vi "LoadControlPanel.vi"(8 "error in (no error)":errorcluster, 10 "Actor In":refnum<class "Actor.lvclass">, 11 "Microscope in":refnum<class "Microscope.lvclass">) -> (0 "error out":errorcluster, 3 "Microscope out":refnum<class "Microscope.lvclass">)   [LabVIEW 2020, in "Microscope.lvlib" / "Microscope.lvclass"]
uses:
  Microscope.lvclass
  <vilib>/ActorFramework/Actor/Actor.lvclass
  Component/Device/Device/DataExchange.ctl
  ViewController/Microscope Controller/MicroscopeController.lvclass
  C:/Program Files/National Instruments/LabVIEW 2020/vi.lib/ActorFramework/Actor/Actor.lvclass
  Microscope.lvclass/Microscope.ctl
  Interface/DataListener Messages/OnDataChange Msg/OnDataChange Msg.lvclass/OnDataChange Msg.ctl
  <vilib>/ActorFramework/Message Enqueuer/Message Enqueuer.lvclass/Message Enqueuer.ctl
  <vilib>/ActorFramework/Message Enqueuer/Enqueue.vi
  Interface/DataListener Messages/OnDataChange Msg/OnDataChange Msg.lvclass
  C:/Program Files/National Instruments/LabVIEW 2020/vi.lib/ActorFramework/Message/Message.lvclass
  <vilib>/ActorFramework/Message Priority Queue/Priority Enqueue.vi
  Component/Device/Device/Device.lvclass
  Interface/DataListener/DataListener.lvclass
panel:
  in  "cluster":T1
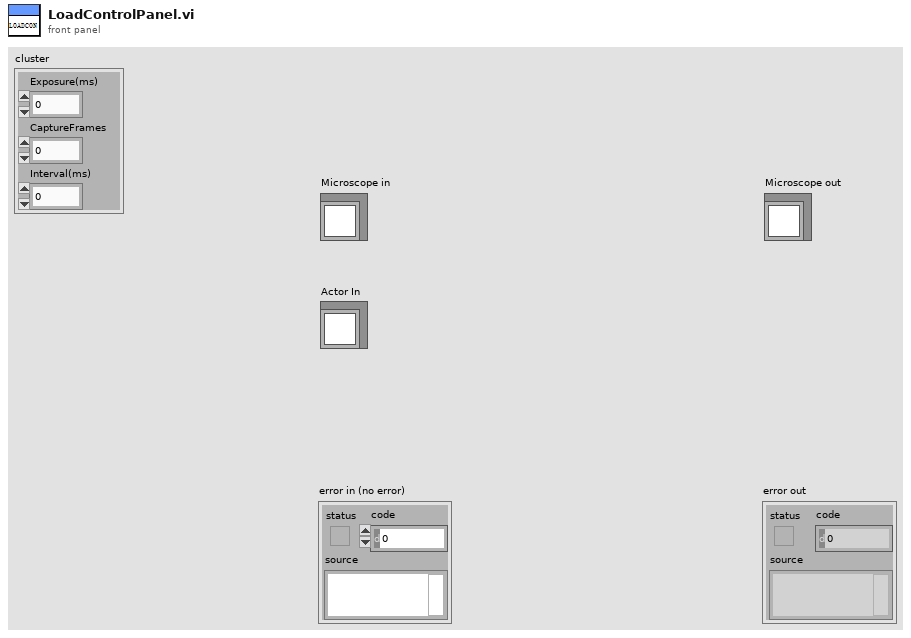
[diagram p1: front panel]
types:
  T1 = cluster{"Exposure(ms)":dbl, "CaptureFrames":dbl, "Interval(ms)":dbl}
  T2 = typedef "DataListener.lvclass/DataExchange.ctl" = cluster{"Source":string, "Destination":string, "Description":string, "value":variant}
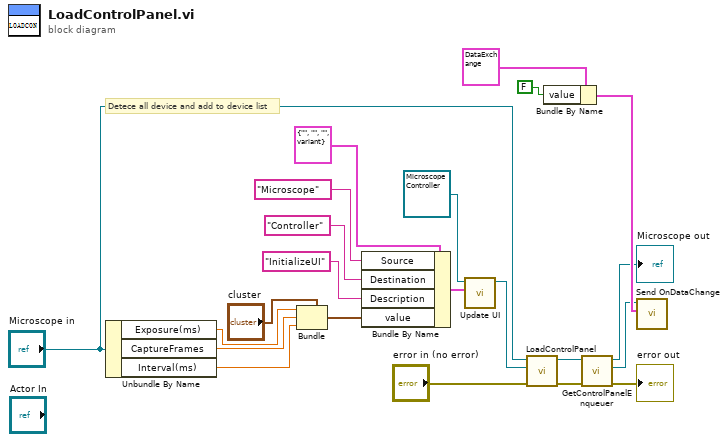
[diagram p0: block diagram]
diagram:
  # "Detece all device and add to device list"
  n1 = Unbundle By Name("Microscope in") -> ("Exposure(ms)"=w8:dbl, "CaptureFrames"=w7:dbl, "Interval(ms)"=w6:dbl)
  n2 = Bundle(cluster="cluster", "Exposure(ms)"=w8, "CaptureFrames"=w7, "Interval(ms)"=w6) -> (w4:T1)
  n3 = Bundle By Name(cluster=T2 {"Source"="", "Destination"="", "Description"="", "value"=variant} ("DataExchange"), "Source"="Microscope", "Destination"="Controller", "Description"="InitializeUI", "value"=w4) -> (w12:T2)
  n4 = call "Update UI.vi"("DataExchange"=w12, "Microscope Controller in"=refnum<class "MicroscopeController.lvclass"> refnum ("MicroscopeController.lvlib:MicroscopeController.lvclass")) -> ("Microscope Controller out"=w2:refnum<class "MicroscopeController.lvclass">)  [unwired: 8 in, 1 out]
  n5 = call-parent "LoadControlPanel.vi"("error in (no error)"="error in (no error)", "Actor In"=w2, "GRMActor in"="Microscope in") -> ("error out"=w22:errorcluster, "GRMActor out"=w16:refnum<class "Microscope.lvclass">)  [unwired: 7 in]
  n6 = Bundle By Name(cluster=T2 {"Source"="Microscope", "Destination"="Bool", "Description"="ShowUI", "value"=variant} ("DataExchange"), "value"=FALSE) -> (w19:T2)
  n7 = call-dynamic "GetControlPanelEnqueuer.vi"("error in (no error)"=w22, "GRMActor in"=w16) -> ("error out"=→"error out":errorcluster, "ControlViewEnqueuer"=w14:refnum<class "Message Enqueuer.lvclass">, "GRMActor out"=→"Microscope out":refnum<class "Microscope.lvclass">)  [unwired: 7 in]
  n8 = call "Send OnDataChange.vi"("DataExchange"=w19, "Message Enqueuer"=w14) -> ()  [unwired: 8 in, 2 out]
